vi "Array Height.vi"(8 "error in (no error)":errorcluster caption="entrée d'erreur (pas d'erreur)", 11 "Acq Cam Basler en entrée":refnum<class "Acq Cam Basler.lvclass">) -> (0 "error out":errorcluster caption="sortie d'erreur", 3 "Acq Cam Basler en sortie":refnum<class "Acq Cam Basler.lvclass">)   [LabVIEW 2023, in "Acq Cam Basler.lvclass"]
uses:
  Acq Cam Basler.lvclass
  Acq Cam Basler.lvclass/Acq Cam Basler.ctl
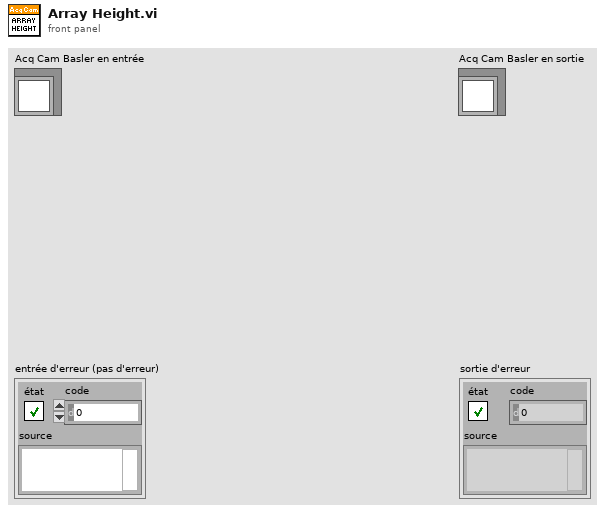
[diagram p1: front panel]
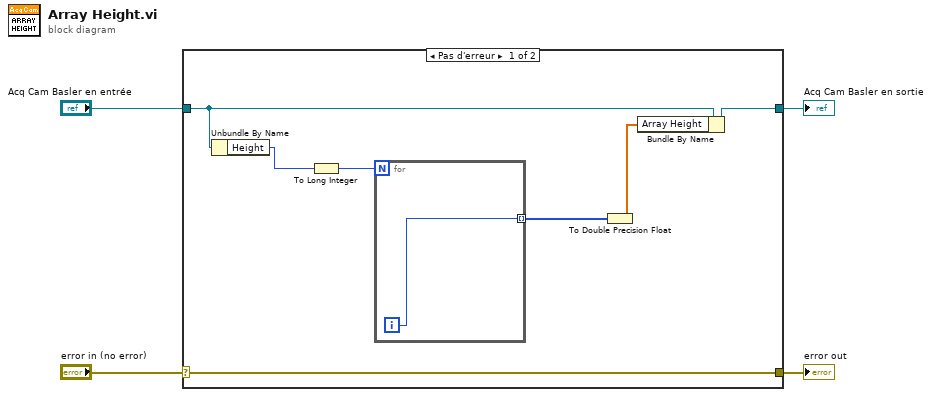
[diagram p0: block diagram]
diagram:
  n1 = case shown="Pas d'erreur" "error in (no error)" {
    selector: "error in (no error)" -> [w11 w14]
    tunnel: [w11 w14] -> w3
    tunnel: [w6 w13] -> w1
    tunnel: "Acq Cam Basler en entrée" -> [w10 w13]
    frame No Error {
      n2 = Unbundle By Name(w10) -> ("Height"=w9:u32)
      n3 = To Long Integer(number=w9) -> (32bit integer=w8:i32)
      n4 = for {
        N: w8 -> [_]
        tunnel: [w12] -> w7 mode=indexing
        i -> [w12]
      }
      n5 = To Double Precision Float(number=w7) -> (double precision float=w5:dbl[])
      n6 = Bundle By Name(cluster=w10, "Array Height"=w5) -> (w6:refnum<class "Acq Cam Basler.lvclass">)
    }
    frame Error {
    }
  }
  "error out" <- w3
  "Acq Cam Basler en sortie" <- w1
